vi "ROI entry-Dynamic obtain Z index.vi"(8 "error in (no error)":errorcluster, 11 "Coordinates":i32[](array[numeric])) -> (0 "error out":errorcluster, 3 "Z-plane selector (index)":i32)   [LabVIEW 2013]
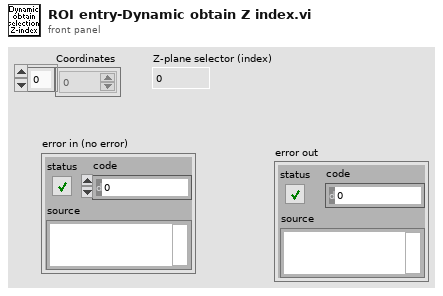
[diagram p1: front panel]
types:
  T1 = typedef "IMAQ Image.ctl" = refnum<image>
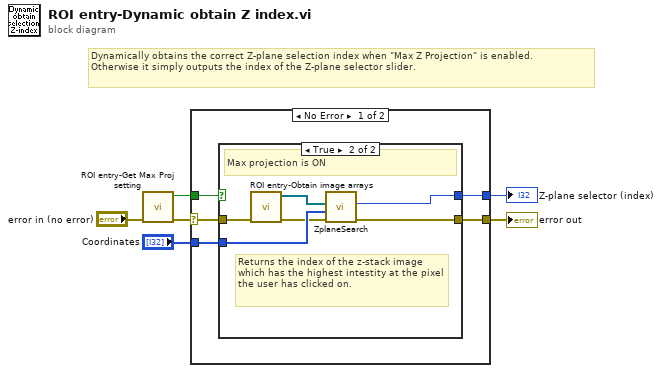
[diagram p0: block diagram]
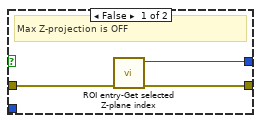
[diagram p2: hidden frame]
diagram:
  # "Dynamically obtains the correct Z-plane selection index when \"Max Z Projection\" is enabled.\nOtherwise it simply outputs the index of the Z-plane selector slider."
  n1 = call "ROI entry-Get Max Proj setting.vi"("error in (no error)"="error in (no error)") -> ("error out"=w2:errorcluster, "Max Z-projection setting's value"=w3:bool)  [unwired: 9 in]
  n2 = case shown="No Error" w2 {
    selector: w2 -> [w7 w21]
    tunnel: "Coordinates" -> [w11 _]
    tunnel: w3 -> [w10 _]
    tunnel: [w9 _] -> w5
    tunnel: [w8 w21] -> w4
    frame No Error {
      n3 = case shown="True" w10 {
        tunnel: w11 -> [_ w19]
        tunnel: [w14 w18] -> w9
        tunnel: w7 -> [w13 w17]
        tunnel: [w12 w15] -> w8
        frame False {
          # "Max Z-projection is OFF"
          n4 = call "ROI entry-Get selected Z-plane index.vi"("error in (no error)"=w13) -> ("error out"=w12:errorcluster, "Z-plane selector (index)"=w14:i32)  [unwired: 9 in]
        }
        frame True {
          # "Returns the index of the z-stack image which has the highest intestity at the pixel the user has clicked on."
          # "Max projection is ON"
          n5 = call "ROI entry-Obtain image arrays.vi"("error in (no error)"=w17) -> ("error IO"=w16:errorcluster, "RedImageArray"=w20:T1[])  [unwired: 9 in]
          n6 = call "ZplaneSearch.vi"("error in (no error)"=w16, "POI"=w19, "ImageArray"=w20) -> ("error out"=w15:errorcluster, "ZplaneIndex"=w18:i32)  [unwired: 7 in]
        }
      }
    }
    frame Error {
    }
  }
  "Z-plane selector (index)" <- w5
  "error out" <- w4
